vi "Read Async Method Error.vi"(8 "error in (no error)":errorcluster, 11 "Async Message in":refnum<class "Async Message.lvclass">) -> (0 "error out":errorcluster, 2 "Async Method Error":errorcluster, 3 "Async Message out":refnum<class "Async Message.lvclass">)   [LabVIEW 2023, in "Async Methods Actor.lvlib" / "Async Message.lvclass"]
uses:
  Async Message.lvclass
  Async Message.lvclass/Async Message.ctl
  Completion Notification Msg/Completion Notification Msg.lvclass/Completion Notification Msg.ctl
  Completion Notification Msg/Completion Notification Msg.lvclass
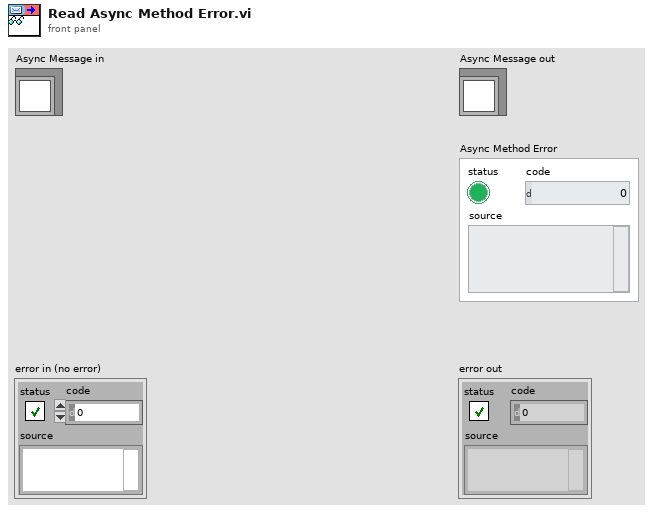
[diagram p1: front panel]
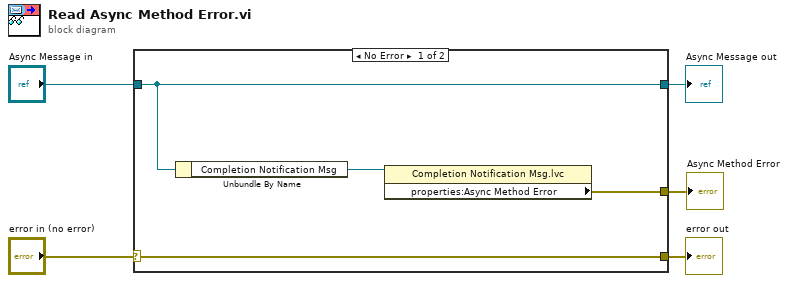
[diagram p0: block diagram]
diagram:
  n1 = case shown="No Error" "error in (no error)" {
    selector: "error in (no error)" -> [w9 w10]
    tunnel: [w9 w10] -> w4
    tunnel: [w8 w11] -> w2
    tunnel: "Async Message in" -> [w8 w11]
    tunnel: [w6 _] -> w1
    frame No Error {
      n2 = Unbundle By Name(w8) -> ("Completion Notification Msg"=w7:refnum<class "Completion Notification Msg.lvclass">)
      n3 = property class="Completion Notification Msg.lvc"(reference=w7) -> ("properties:Async Method Error"=w6:errorcluster)  [unwired: 1 in, 2 out]
    }
    frame Error {
    }
  }
  "error out" <- w4
  "Async Message out" <- w2
  "Async Method Error" <- w1
